vi "serverstreaming_client.vi"() -> ()   [LabVIEW 2019]
uses:
  Generated_client/RPC Messages/Request.ctl
  Generated_client/RPC Messages/Request_request_oneof/Request_request_oneof.lvclass
  Generated_client/RPC Messages/Request_request_oneof/Request_request_oneof.lvclass/Request_request_oneof.ctl
  Generated_client/RPC Messages/Response_response_oneof/Response_response_oneof.lvclass/Response_response_oneof.ctl
  Generated_client/Generated_client.lvlib
  Generated_client/RPC Messages/Response_response_oneof/Response_response_oneof.lvclass
panel:
  out "error out":errorcluster
  out "results":string[](array[string])
  out "resp_id":i32[](array[numeric])
  out "new_age":i32[](array[numeric])
  in  "age":i32
  in  "req_id":i32
  in  "message":string
  in  "req_oneof":enum16{"message", "req_id"}(ring)
  in  "error in":errorcluster
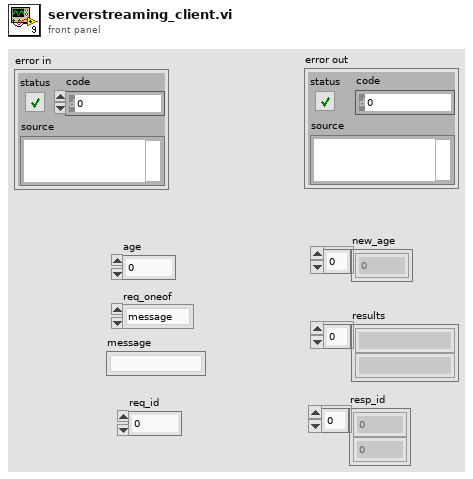
[diagram p1: front panel]
types:
  T1 = typedef "Generated_client.lvlib/Request.ctl" = cluster{"age":i32, "Request_request_oneof":refnum<class "Request_request_oneof.lvclass">}
  T2 = typedef "grpc-lvsupport-release.lvlib/grpcId.ctl" = u64
  T3 = typedef "Generated_client.lvlib/Response.ctl" = cluster{"new_age":i32, "Response_response_oneof":refnum<class "Response_response_oneof.lvclass">}
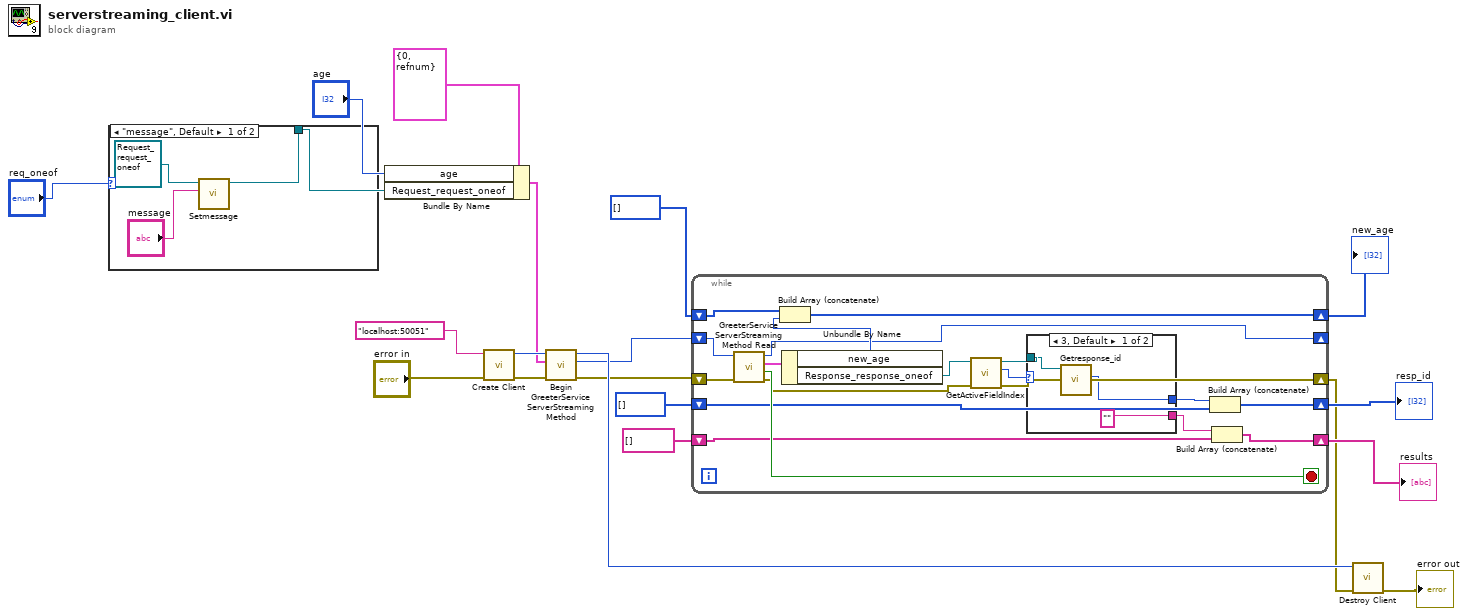
[diagram p0: block diagram]
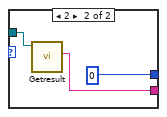
[diagram p2: hidden frame]
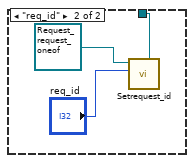
[diagram p3: hidden frame]
diagram:
  n1 = case shown="\"message\", Default" "req_oneof" {
    tunnel: [w21 w24] -> w16
    frame "message", Default {
      n2 = call "Setmessage.vi"("Set_Val"="message", "OneOfTemplate in"=refnum<class "Request_request_oneof.lvclass"> refnum) -> ("OneOfTemplate out"=w21:refnum<class "Request_request_oneof.lvclass">)  [unwired: 8 in, 1 out]
    }
    frame "req_id" {
      n3 = call "Setrequest_id.vi"("Set_Val"="req_id", "OneOfTemplate in"=refnum<class "Request_request_oneof.lvclass"> refnum) -> ("OneOfTemplate out"=w24:refnum<class "Request_request_oneof.lvclass">)  [unwired: 8 in, 1 out]
    }
  }
  n4 = Bundle By Name(cluster=T1 {"age"=0, "Request_request_oneof"=refnum} ("Request"), "age"="age", "Request_request_oneof"=w16) -> (w12:T1)
  n5 = call "Create Client.vi"("error in"="error in", "address"="localhost:50051") -> ("error out"=w13:errorcluster, "gRPC ID Out"=w14:T2)  [unwired: 8 in]
  n6 = call "Begin GreeterService ServerStreamingMethod.vi"("error in"=w13, "Request Data"=w12, "gRPC ID"=w14) -> ("error out"=w10:errorcluster, "Call Id Out"=w2:T2, "gRPC ID out"=w11:T2)  [unwired: 6 in]
  n7 = while {
    shift-right: [w29] -> w1
    shift-left: w10 -> [w45]
    shift-right: [w41] -> w6
    shift-left: i32[] [] -> [w42]
    shift-right: [w34] -> w4
    shift-left: string[] [] -> [w35]
    shift-right: [w31] -> w5
    shift-left: i32[] [] -> [w32]
    shift-right: [w27] -> _
    shift-left: w2 -> [w28]
    stop <- w37 stop-if-true
    n8 = call "GreeterService ServerStreamingMethod Read.vi"("error in"=w45, "Call ID in"=w28) -> ("error out"=w30:errorcluster, "Success"=w37:bool, "Response Data"=w44:T3, "Call ID"=w27:T2)  [unwired: 6 in]
    n9 = Unbundle By Name(w44) -> ("new_age"=w43:i32, "Response_response_oneof"=w40:refnum<class "Response_response_oneof.lvclass">)
    n10 = Build Array (concatenate)(w42, w43) -> (w41:i32[])
    n11 = call "GetActiveFieldIndex.vi"("error in (no error)"=w30, "OneOfTemplate in"=w40) -> ("error out"=w29:errorcluster, "Active Field Index"=w39:i32, "OneOfTemplate out"=w38:refnum<class "Response_response_oneof.lvclass">)  [unwired: 7 in]
    n12 = case shown="3, Default" w39 {
      tunnel: w38 -> [w48 w51]
      tunnel: ["" ("Get_Val") w50] -> w36
      tunnel: [w47 0 ("Get_Val")] -> w33
      frame 3, Default {
        n13 = call "Getresponse_id.vi"("OneOfTemplate in"=w48) -> ("Get_Val"=w47:i32)  [unwired: 8 in, 2 out]
      }
      frame 2 {
        n14 = call "Getresult.vi"("OneOfTemplate in"=w51) -> ("Get_Val"=w50:string)  [unwired: 8 in, 2 out]
      }
    }
    n15 = Build Array (concatenate)(w33, w32) -> (w31:i32[])
    n16 = Build Array (concatenate)(w36, w35) -> (w34:string[])
  }
  "new_age" <- w6
  "resp_id" <- w5
  "results" <- w4
  n17 = call "Destroy Client.vi"("error in"=w1, "gRPC ID"=w11) -> ("error out"=→"error out":errorcluster)  [unwired: 9 in]
